vi "Run Bfr Rx - PingPongSized - Add to Active.vi"(5 "Data Size in":u64, 7 "Data in":u8[](array[numeric]), 8 "error in (no error)":errorcluster, 11 "Ping Pong Buffer in":T1 {"Active Buffer Ref" format="%016x"}) -> (0 "error out":errorcluster, 3 "Ping Pong Buffer out":T1 {"Active Buffer Ref" format="%016x"})   [LabVIEW 2016, in "UDP-Custom-Device Engine.lvlib"]
uses:
  UDP-Custom-Device Engine.lvlib
  Types/Engine - Buffered Rx Ping Pong Buffer.ctl
  Types/Engine - Buffered Rx Active Buffer.ctl
  <vilib>/NI Veristand/VeriStand Data/Pointer Operations/Pointer.Write (I32).vi
  <vilib>/NI Veristand/VeriStand Data/Pointer Operations/Pointer.Read (U16).vi
  <vilib>/NI Veristand/VeriStand Data/Pointer Operations/Pointer.Write (U16).vi
  <vilib>/NI Veristand/VeriStand Data/Pointer Operations/Pointer.Write (1D U8).vi
  <vilib>/NI Veristand/VeriStand Data/Pointer Operations/Pointer.In-Place Read (U16).vi
  <vilib>/NI Veristand/VeriStand Data/VeriStand Data.lvlib
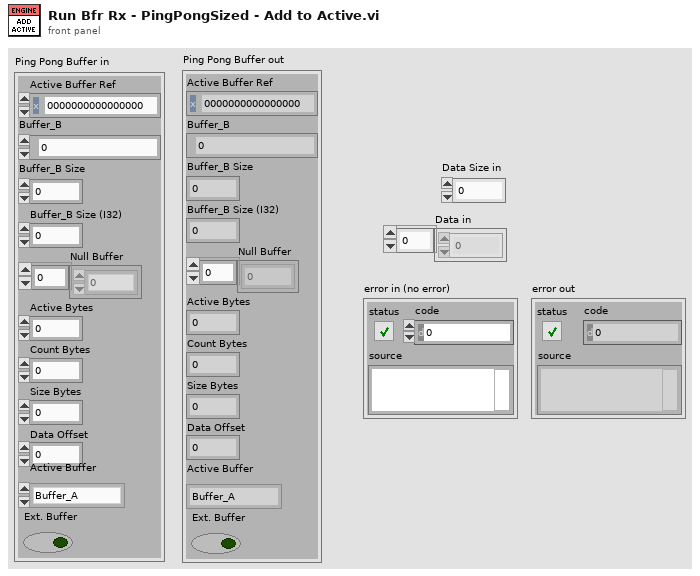
[diagram p1: front panel]
types:
  T1 = typedef "UDP-Custom-Device Engine.lvlib/Engine - Buffered Rx Ping Pong Buffer.ctl" = cluster{"Active Buffer Ref":u64, "Buffer_B":u64, "Buffer_B Size":u64, "Buffer_B Size (I32)":i32, "Null Buffer":u8[], "Active Bytes":u64, "Count Bytes":u64, "Size Bytes":u64, "Data Offset":u64, "Active Buffer":T2, "Ext. Buffer":bool}
  T2 = typedef "UDP-Custom-Device Engine.lvlib/Engine - Buffered Rx Active Buffer.ctl" = enum16{"Buffer_A", "Buffer_B"}
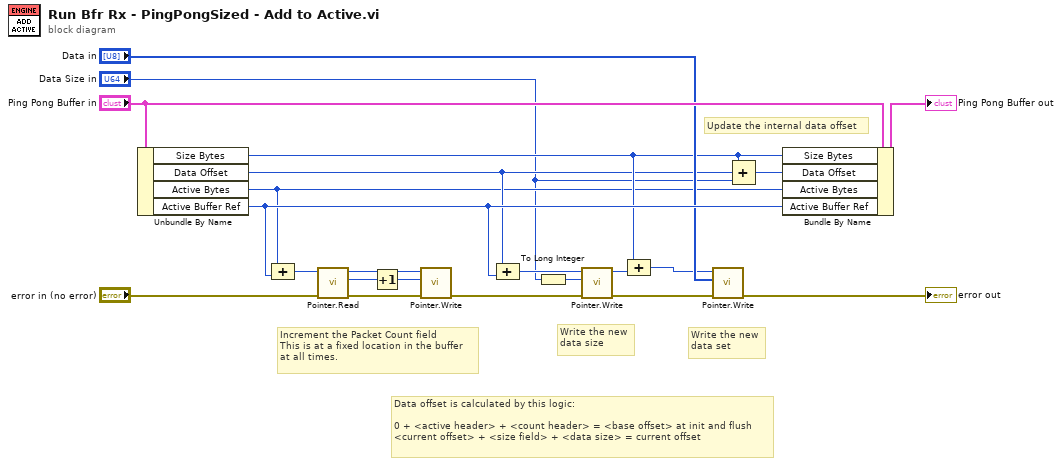
[diagram p0: block diagram]
diagram:
  # "Data offset is calculated by this logic:\n\n0 + <active header> + <count header> = <base offset> at init and flush\n<current offset> + <size field> + <data size> = current offset"
  # "Write the new\ndata set"
  # "Write the new\ndata size"
  # "Increment the Packet Count field\nThis is at a fixed location in the buffer\nat all times."
  # "Update the internal data offset"
  n1 = Unbundle By Name("Ping Pong Buffer in") -> ("Size Bytes"=w5:u64, "Data Offset"=w4:u64, "Active Bytes"=w3:u64, "Active Buffer Ref"=w9:u64)
  n2 = Compound Arithmetic op=ADD(w3, w9) -> (w16:u64)
  n3 = call-poly <vilib>:"Pointer.Read.vi"("error in (no error)"="error in (no error)", "pointer in"=w16) -> ("error out"=w17:errorcluster, "value"=w19:u16, "pointer out"=w18:u64)  [unwired: 7 in]
  n4 = Increment(x=w19) -> (x+1=w20:u16)
  n5 = call-poly <vilib>:"Pointer.Write.vi"("error in (no error)"=w17, "value"=w20, "pointer in"=w18) -> ("error out"=w14:errorcluster)  [unwired: 6 in, 2 out]
  n6 = Compound Arithmetic op=ADD(w4, w9) -> (w10:u64)
  n7 = To Long Integer(number="Data Size in") -> (32bit integer=w11:i32)
  n8 = call-poly <vilib>:"Pointer.Write.vi"("error in (no error)"=w14, "value"=w11, "pointer in"=w10) -> ("error out"=w13:errorcluster, "pointer out"=w7:u64)  [unwired: 6 in, 1 out]
  n9 = Compound Arithmetic op=ADD(w5, w7) -> (w6:u64)
  n10 = call-poly <vilib>:"Pointer.Write.vi"("error in (no error)"=w13, "values"="Data in", "pointer in"=w6) -> ("error out"=→"error out":errorcluster)  [unwired: 6 in, 2 out]
  n11 = Compound Arithmetic op=ADD(w5, w4, "Data Size in") -> (w1:u64)
  n12 = Bundle By Name(cluster="Ping Pong Buffer in", "Size Bytes"=w5, "Data Offset"=w1, "Active Bytes"=w3, "Active Buffer Ref"=w9) -> (→"Ping Pong Buffer out":T1)
